vi "ConvertU64ToLVDBL.vi"(4 "Time U64 LowPart":u32, 5 "Time U64 HighPart":u32) -> (1 "Time LV DBL":dbl format="%.2f")   [LabVIEW 2016]
doc: "Convert from U64 100ns intervals since Jan 1 1601 GMT (Win32 FILETIME) to DBL seconds since Jan 1 1904 GMT (LabVIEW DBL time)"
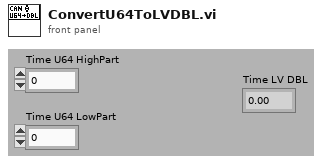
[diagram p1: front panel]
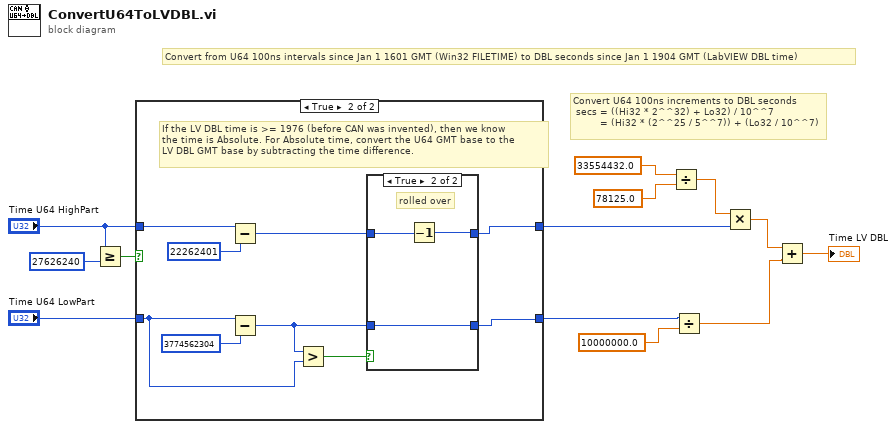
[diagram p0: block diagram]
diagram:
  # "Convert U64 100ns increments to DBL seconds\n secs = ((Hi32 * 2^^32) + Lo32) / 10^^7\n         = (Hi32 * (2^^25 / 5^^7)) + (Lo32 / 10^^7)"
  # "Convert from U64 100ns intervals since Jan 1 1601 GMT (Win32 FILETIME) to DBL seconds since Jan 1 1904 GMT (LabVIEW DBL time)"
  n1 = Greater Or Equal?(x="Time U64 HighPart", y=u32 27626240) -> (x >= y?=w12:bool)
  n2 = case shown="True" w12 {
    tunnel: "Time U64 HighPart" -> [w15 w22]
    tunnel: "Time U64 LowPart" -> [w14 w21]
    tunnel: [w15 w16] -> w5
    tunnel: [w14 w18] -> w9
    frame False {
      # "If the U64 time is less than 1976, then we know the time is Relative.\nThe Rekative maximum allows for more than 73 years of continuous\nacquisition/logging."
    }
    frame True {
      # "If the LV DBL time is >= 1976 (before CAN was invented), then we know \nthe time is Absolute. For Absolute time, convert the U64 GMT base to the \nLV DBL GMT base by subtracting the time difference."
      n3 = Subtract(x=w22, y=u32 22262401) -> (x-y=w17:u32)
      n4 = Subtract(x=w21, y=u32 3774562304) -> (x-y=w19:u32)
      n5 = Greater?(x=w19, y=w21) -> (0:w20:bool)
      n6 = case shown="True" w20 {
        tunnel: w19 -> [w26 w29]
        tunnel: [w26 w29] -> w18
        tunnel: [w25 w27] -> w16
        tunnel: w17 -> [w25 w28]
        frame False {
        }
        frame True {
          # "rolled over"
          n7 = Decrement(x=w28) -> (x-1=w27:u32)
        }
      }
    }
  }
  n8 = Divide(x=33554432.0, y=78125.0) -> (x/y=w4:dbl)
  n9 = Divide(x=w9, y=10000000.0) -> (x/y=w2:dbl)
  n10 = Multiply(x=w4, y=w5) -> (x*y=w3:dbl)
  n11 = Add(x=w3, y=w2) -> (x+y=→"Time LV DBL":dbl)
